vi "Utility - Configuration File Generator- Waveform _V1.2.vi"() -> ()   [LabVIEW 2015]
uses:
  <vilib>/LabVIEW Targets/FPGA/cRIO/shared/nicrio_ModuleControls/nicrio_cRIO-9234_DataRatesRing2.ctl
  TDMS Properties.ctl
  <vilib>/LabVIEW Targets/FPGA/cRIO/shared/nicrio_ModuleControls/nicrio_cRIO-9234_ConfigModeRing.ctl
  STA - Waveform V6/Config/Data Rate Conversion.ctl
  Acquisition and Logging Configuration_Waveform - V1.ctl
  <vilib>/Utility/xml.llb/Write to XML File(string).vi
panel:
  out "unsigned 32bit integer":u32
  out "appended path 2":path
  out "appended path":path
  in  "Data Rate Conversion":T1=[51200.0, 25600.0, 17067.0, 12800.0, 10240.0, 8533.0, 7314.0, 6400.0, 5689.0, 5120.0, 4654.0, 4267.0, 3938.0, 3657.0, 3413.0, 3200.0, 3012.0, 2845.0, 2695.0, 2560.0, 2438.0, 2328.0, 2226.0, 2133.0, 2048.0, 1969.0, 1896.0, 1829.0, 1765.0, 1707.0, 1652.0]
  in  "Firt raw Config repeat?":bool
  in  "Time Measure (s)":dbl=60.0
  in  "Channel Config":T3(array[cluster])=[{"Channel Name"="mod1/a0\na0\na00\na00", "Sensitivity mV_EU"=1.016, "EU"="ms²", "Input Configuration"=0, "dB Ref EU"=1.0}, {"Channel Name"="mod1/a1", "Sensitivity mV_EU"=1.0, "EU"="V", "Input Configuration"=0, "dB Ref EU"=1.0}, {"Channel Name"="mod1/a2", "Sensitivity mV_EU"=1.0, "EU"="V", "Input Configuration"=0, "dB Ref EU"=1.0}, {"Channel Name"="mod1/a3", "Sensitivity mV_EU"=1.0, "EU"="V", "Input Configuration"=0, "dB Ref EU"=1.0}, {"Channel Name"="mod2/a0", "Sensitivity mV_EU"=1000.0, "EU"="V", "Input Configuration"=0, "dB Ref EU"=1.0}, {"Channel Name"="mod2/a1", "Sensitivity mV_EU"=1000.0, "EU"="V", "Input Configuration"=0, "dB Ref EU"=1.0}, {"Channel Name"="mod2/a2", "Sensitivity mV_EU"=1000.0, "EU"="V", "Input Configuration"=0, "dB Ref EU"=1.0}, {"Channel Name"="mod2/a3", "Sensitivity mV_EU"=1000.0, "EU"="V", "Input Configuration"=0, "dB Ref EU"=1.0}, {"Channel Name"="mod3/a0", "Sensitivity mV_EU"=1000.0, "EU"="V", "Input Configuration"=0, "dB Ref EU"=1.0}, {"Channel Name"="mod3/a1", "Sensitivity mV_EU"=1000.0, "EU"="V", "Input Configuration"=0, "dB Ref EU"=1.0}, {"Channel Name"="mod3/a2", "Sensitivity mV_EU"=1000.0, "EU"="V", "Input Configuration"=0, "dB Ref EU"=1.0}, {"Channel Name"="mod3/a3", "Sensitivity mV_EU"=1000.0, "EU"="V", "Input Configuration"=0, "dB Ref EU"=1.0}, {"Channel Name"="mod4/a0", "Sensitivity mV_EU"=1000.0, "EU"="V", "Input Configuration"=0, "dB Ref EU"=1.0}, {"Channel Name"="mod4/a1", "Sensitivity mV_EU"=1000.0, "EU"="V", "Input Configuration"=0, "dB Ref EU"=1.0}, {"Channel Name"="mod4/a2", "Sensitivity mV_EU"=1000.0, "EU"="V", "Input Configuration"=0, "dB Ref EU"=1.0}, {"Channel Name"="mod4/a3", "Sensitivity mV_EU"=1000.0, "EU"="V", "Input Configuration"=0, "dB Ref EU"=1.0}] caption="Channel Name      Sensitivity [mV/EU]              EU                           dB Ref [EU]                Input Typ" {"Input Configuration" items=["AC Coupled", "DC Coupled", "IEPE AC Coupled"]}
  in  "TDMS Properties":T4[](array[typedef])=[{"Name"="Enterprise", "Value"="[CompanyName]"}, {"Name"="Author", "Value"="[DeveloperName]"}, {"Name"="Operator", "Value"="[OperatorName]"}, {"Name"="TestSystem", "Value"="[SystemName]"}, {"Name"="Site", "Value"="[Location]"}, {"Name"="Line", "Value"="[Line]"}, {"Name"="Machine", "Value"="[MachineName]"}, {"Name"="Description", "Value"="[Description]"}]
  in  "Trigger - Time (Minute)":i32=30
  in  "Trigger - Channel":i32
  in  "Trigger - RMS Value":dbl=1.8
  in  "Number of Channels":i32=16
  in  "Data File Name":string="cRIO_Data"
  in  "Samples per Read":i32=12800
  in  "Data Rate":T5=1 items=["51.200 kS/s (NI 9234)"=1, "25.600 kS/s (NI 9234)"=2, "17.067 kS/s (NI 9234)"=3, "12.800 kS/s (NI 9234)"=4, "10.240 kS/s (NI 9234)"=5, "8.533 kS/s (NI 9234)"=6, "7.314 kS/s (NI 9234)"=7, "6.400 kS/s (NI 9234)"=8, "5.689 kS/s (NI 9234)"=9, "5.120 kS/s (NI 9234)"=10, "4.654 kS/s (NI 9234)"=11, "4.267 kS/s (NI 9234)"=12, "3.938 kS/s (NI 9234)"=13, "3.657 kS/s (NI 9234)"=14, "3.413 kS/s (NI 9234)"=15, "3.200 kS/s (NI 9234)"=16, "3.012 kS/s (NI 9234)"=17, "2.845 kS/s (NI 9234)"=18, "2.695 kS/s (NI 9234)"=19, "2.560 kS/s (NI 9234)"=20, "2.438 kS/s (NI 9234)"=21, "2.328 kS/s (NI 9234)"=22, "2.226 kS/s (NI 9234)"=23, "2.133 kS/s (NI 9234)"=24, "2.048 kS/s (NI 9234)"=25, "1.969 kS/s (NI 9234)"=26, "1.896 kS/s (NI 9234)"=27, "1.829 kS/s (NI 9234)"=28, "1.765 kS/s (NI 9234)"=29, "1.707 kS/s (NI 9234)"=30, "1.652 kS/s (NI 9234)"=31]
  # "Instructions: Populate the controls below with desired values, then run the VI to generate a 'Config.xml' file in the root folder of your project.  \n\nNote:  Once you have generated the Config.xml file, you will need to copy it to the root folder of your RT Target."
  # "Acquisition"
  # "Logging"
  # "Channels"
  # "Trigger"
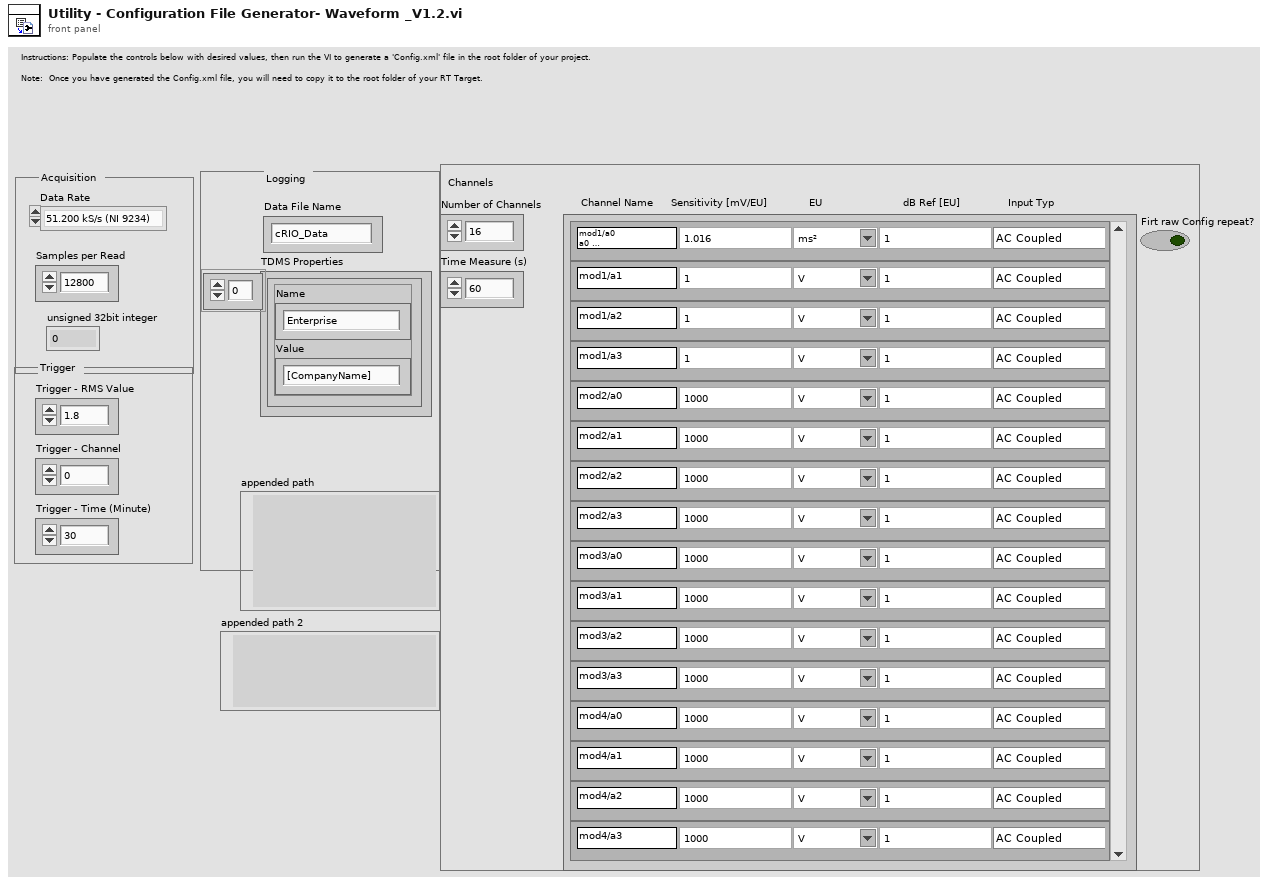
[diagram p1: front panel]
types:
  T1 = typedef "Data Rate Conversion.ctl" = dbl[]
  T2 = typedef "nicrio_cRIO-9234_ConfigModeRing.ctl" = u8
  T3 = cluster{"Channel Name":string, "Sensitivity mV_EU":dbl, "EU":string, "Input Configuration":T2, "dB Ref EU":dbl}[]
  T4 = typedef "TDMS Properties.ctl" = cluster{"Name":string, "Value":string}
  T5 = typedef "nicrio_cRIO-9234_DataRatesRing2.ctl" = u8
  T6 = typedef "Acquisition and Logging Configuration_Waveform - V1.ctl" = cluster{"Samples per Read":i32, "Number of Reads to Save":i32, "Data File Name":string, "TDMS Properties":T4[], "Number of Channels":i32, "Trigger - RMS Value":dbl, "Trigger - Channel":i32, "Trigger - Time (Minute)":i32, "Channel Config":cluster{"Channel Name":string, "Sensitivity mV_EU":dbl, "EU":string, "Input Configuration":T2, "dB Ref EU":dbl}[], "data rate (S/s)":u32, "Time Measure":dbl}
  T7 = cluster{"Channel Name":string, "Sensitivity mV_EU":dbl, "EU":string, "Input Configuration":T2, "dB Ref EU":dbl}
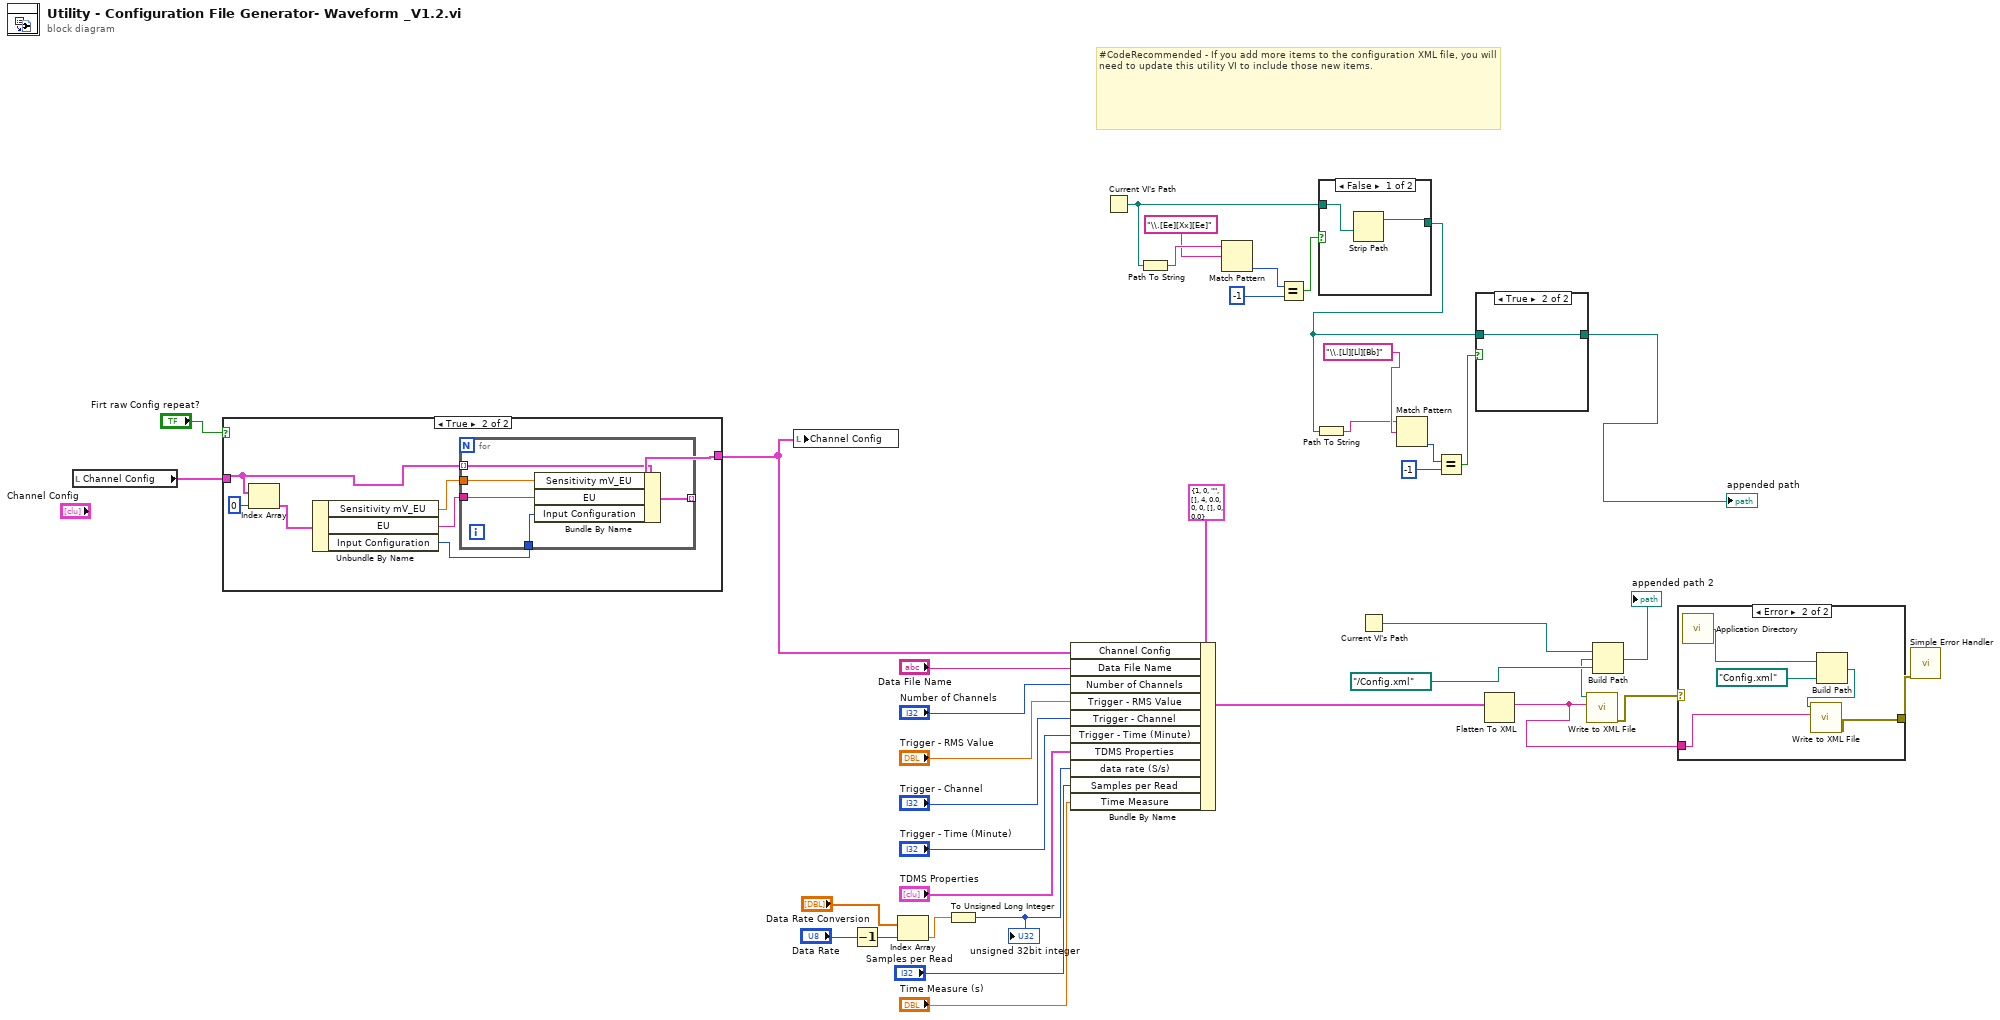
[diagram p0: block diagram]
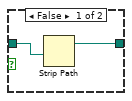
[diagram p4: hidden frame]
diagram:
  # "#CodeRecommended - If you add more items to the configuration XML file, you will need to update this utility VI to include those new items."
  n1 = local read "Channel Config"() -> (w15:T3)
  n2 = case shown="True" "Firt raw Config repeat?" {
    tunnel: w15 -> [w38 w39]
    tunnel: [w38 w40] -> w14
    frame False {
    }
    frame True {
      n3 = Index Array(array=w39, index=0) -> (element=w44:T7)
      n4 = Unbundle By Name(w44) -> ("Sensitivity mV_EU"=w43:dbl, "EU"=w42:string, "Input Configuration"=w41:T2)
      n5 = for {
        tunnel: w39 -> [w46] mode=indexing
        tunnel: w43 -> [w50]
        tunnel: w42 -> [w49]
        tunnel: w41 -> [w48]
        tunnel: [w47] -> w40 mode=indexing
        n6 = Bundle By Name(cluster=w46, "Sensitivity mV_EU"=w50, "EU"=w49, "Input Configuration"=w48) -> (w47:T7)
      }
    }
  }
  n7 = local write "Channel Config"(w14) -> ()
  n8 = Decrement(x="Data Rate") -> (x-1=w12:T5)
  n9 = Index Array(array="Data Rate Conversion", index=w12) -> (element=w11:dbl)
  n10 = To Unsigned Long Integer(number=w11) -> (unsigned 32bit integer=w10:u32)
  "unsigned 32bit integer" <- w10
  n11 = Bundle By Name(cluster=T6 {"Samples per Read"=1, "Number of Reads to Save"=0, "Data File Name"="", "TDMS Properties"=[], "Number of Channels"=4, "Trigger - RMS Value"=0.0, "Trigger - Channel"=0, "Trigger - Time (Minute)"=0, "Channel Config"=[], "data rate (S/s)"=0, "Time Measure"=0.0} ("Acquisition and Logging Configuration"), "Channel Config"=w14, "Data File Name"="Data File Name", "Number of Channels"="Number of Channels", "Trigger - RMS Value"="Trigger - RMS Value", "Trigger - Channel"="Trigger - Channel", "Trigger - Time (Minute)"="Trigger - Time (Minute)", "TDMS Properties"="TDMS Properties", "data rate (S/s)"=w10, "Samples per Read"="Samples per Read", "Time Measure"="Time Measure (s)") -> (w30:T6)
  n12 = Current VI's Path() -> (path=w26:path)
  n13 = Path To String(path=w26) -> (string=w27:string)
  n14 = Match Pattern(string=w27, regular expression="\\.[Ee][Xx][Ee]") -> (offset past match=w18:i32)  [unwired: 1 in, 3 out]
  n15 = Equal?(x=w18, y=-1) -> (x = y?=w28:bool)
  n16 = case shown="False" w28 {
    tunnel: [w52 w53] -> w19
    tunnel: w26 -> [w51 w53]
    frame False {
      n17 = Strip Path(path=w51) -> (stripped path=w52:path)  [unwired: 1 out]
    }
    frame True {
    }
  }
  n18 = Path To String(path=w19) -> (string=w23:string)
  n19 = Current VI's Path() -> (path=w1:path)
  n20 = Match Pattern(string=w23, regular expression="\\.[Ll][Ll][Bb]") -> (offset past match=w20:i32)  [unwired: 1 in, 3 out]
  n21 = Equal?(x=w20, y=-1) -> (x = y?=w22:bool)
  n22 = case shown="True" w22 {
    tunnel: [w55 w56] -> w6
    tunnel: w19 -> [w54 w56]
    frame False {
      n23 = Strip Path(path=w54) -> (stripped path=w55:path)  [unwired: 1 out]
    }
    frame True {
    }
  }
  "appended path" <- w6
  n24 = Flatten To XML(anything=w30) -> (xml string=w3:string)
  n25 = Build Path(base path=w1, name or relative path=path "../Config.xml") -> (appended path=w5:path)
  "appended path 2" <- w5
  n26 = call-poly <vilib>:"Write to XML File.vi"("XML Input"=w3, "XML File Path"=w5) -> ("error out"=w4:errorcluster)  [unwired: 7 in, 2 out]
  n27 = case shown="Error" w4 {
    selector: w4 -> [w57 _]
    tunnel: w3 -> [_ w58]
    tunnel: [w57 w59] -> w2
    frame No Error {
    }
    frame Error {
      n28 = call <vilib>:"Application Directory.vi"() -> ("Application Directory"=w61:path)
      n29 = Build Path(base path=w61, name or relative path=path "Config.xml") -> (appended path=w60:path)
      n30 = call-poly <vilib>:"Write to XML File.vi"("XML Input"=w58, "XML File Path"=w60) -> ("error out"=w59:errorcluster)  [unwired: 7 in, 2 out]
    }
  }
  n31 = call <vilib>:"Simple Error Handler.vi"("error in (no error)"=w2) -> ()  [unwired: 4 in, 5 out]
